vi "Filter Error (1D).vi"(0 "error in (no error)":errorcluster, 1 "Array":i32[](array[numeric])) -> (2 "error out":errorcluster)   [LabVIEW 2020]
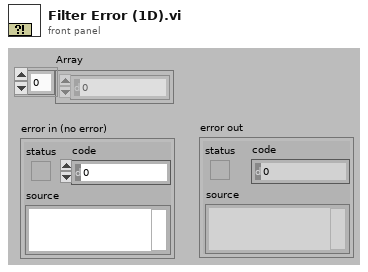
[diagram p1: front panel]
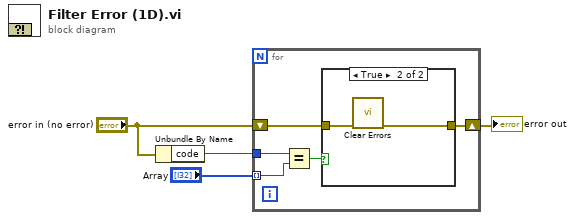
[diagram p0: block diagram]
diagram:
  n1 = Unbundle By Name("error in (no error)") -> ("code"=w4:i32)
  n2 = for {
    tunnel: w4 -> [w9]
    tunnel: "Array" -> [w5] mode=indexing
    shift-right: [w6] -> w2
    shift-left: "error in (no error)" -> [w7]
    n3 = Equal?(x=w9, y=w5) -> (x = y?=w8:bool)
    n4 = case shown="True" w8 {
      tunnel: w7 -> [w10 w12]
      tunnel: [w10 w11] -> w6
      frame False {
      }
      frame True {
        n5 = call <vilib>:"Clear Errors.vi"("error in (no error)"=w12) -> ("error out"=w11:errorcluster)  [unwired: 5 in, 1 out]
      }
    }
  }
  "error out" <- w2
